vi "Marquee.vi"(8 "Indicator or ctrl to look up value change":refnum<vi>, 9 "Iteration":i8, 10 "error in (no error)":errorcluster, 11 "Text":string) -> (2 "error out":errorcluster, 3 "shutdown":bool=TRUE)   [LabVIEW 2021]
doc: "Showing marquee animation"
uses:
  System.Windows.Forms
panel:
  in  "Panel":refnum<k24>(container) caption="Closing WebSDR Cat-Control...."
  in  "stop":bool
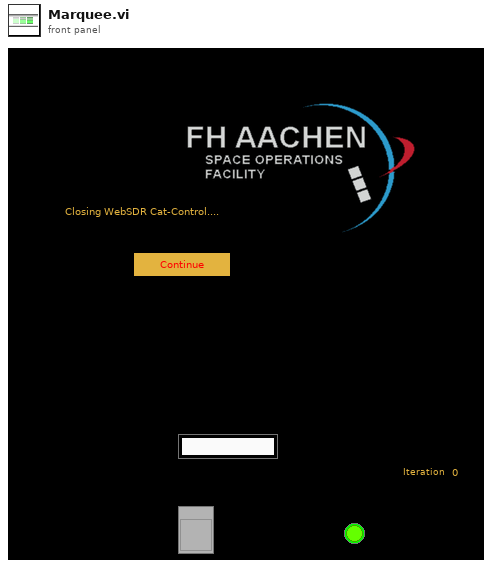
[diagram p1: front panel]
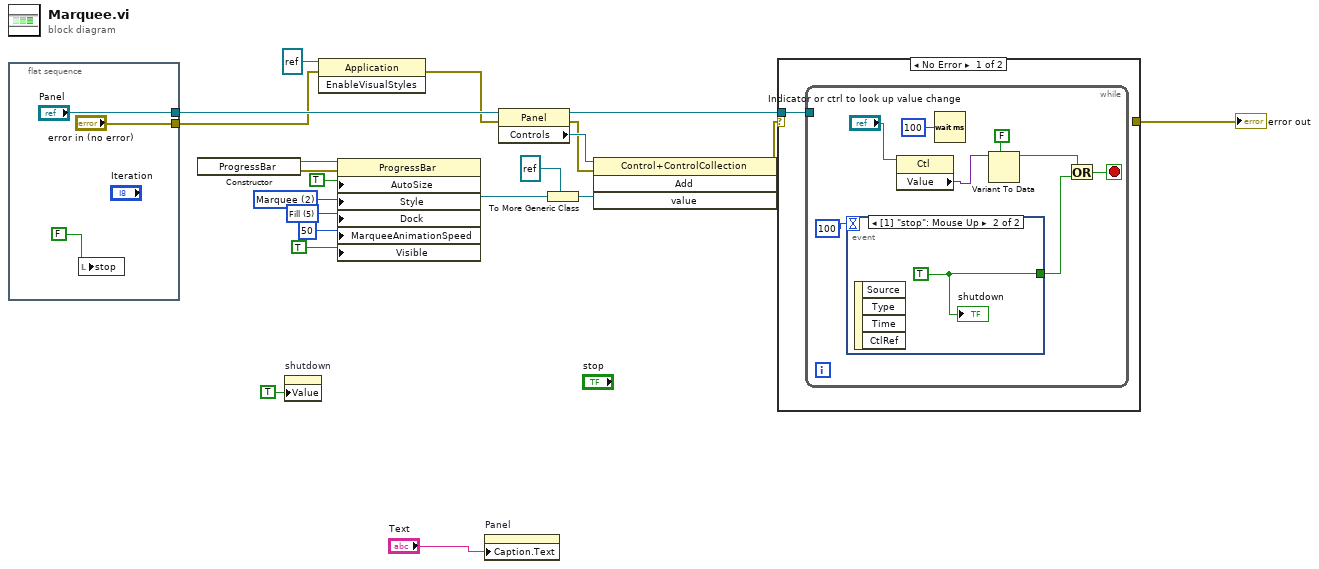
[diagram p0: block diagram]
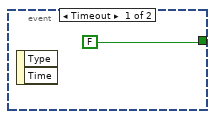
[diagram p2: hidden frame]
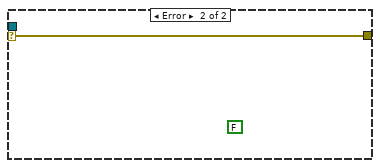
[diagram p3: hidden frame]
diagram:
  w16 = 5 items=["None", "Top", "Bottom", "Left", "Right", "Fill"] ("Dock")
  w15 = 2 items=["Blocks", "Continuous", "Marquee"] ("Style")
  n1 = flat-sequence {
    tunnel: ["Panel"] -> w21
    tunnel: ["error in (no error)"] -> w4
    frame #0 {
      n2 = local write "stop"(FALSE ("ABORT?")) -> ()
    }
  }
  n3 = constructor class="ProgressBar"() -> (reference out=w12:refnum<k24>, error out=w14:errorcluster)  [unwired: 3 in, 1 out]
  n4 = property on="shutdown" class="Bool (strict)"("Value"=TRUE ("shutdown")) -> ()  [unwired: 2 in, 2 out]
  n5 = invoke class="Application" method="EnableVisualStyles"(reference=refnum<k24> refnum ("new reference"), error in=w4) -> (error out=w3:errorcluster)  [unwired: 1 in, 2 out]
  n6 = property class="ProgressBar"(reference=w12, error in=w14, "AutoSize"=TRUE, "Style"=w15, "Dock"=w16, "MarqueeAnimationSpeed"=50, "Visible"=TRUE) -> (reference out=w8:refnum<k24>)  [unwired: 1 out]
  n7 = property on="Panel" class="AXCont"("Caption.Text"="Text") -> ()  [unwired: 2 in, 2 out]
  n8 = property class="Panel"(reference=w21, error in=w3) -> (reference out=w20:refnum<k24>, error out=w7:errorcluster, "Controls"=w11:refnum<k24>)
  n9 = To More Generic Class(target class=refnum<k24> refnum, reference=w8) -> (generic class reference=w9:refnum<k24>)
  n10 = invoke class="Control+ControlCollection" method="Add"(reference=w11, error in=w7, "value"=w9) -> (error out=w6:errorcluster)  [unwired: 1 in, 3 out]
  n11 = case shown="No Error" w6 {
    selector: w6 -> [_ w36]
    tunnel: w20 -> [w25 _]
    tunnel: [_ w36] -> w19
    frame No Error {
      n12 = while {
        tunnel: w25 -> [_]
        stop <- w31 stop-if-true
        n13 = event shown="[1] \"stop\": Mouse Up" {
          selector: _ -> [_ _]
          dyn-events: _ -> [_ _]
          timeout: 100 -> [_ _]
          tunnel: [FALSE w35] -> w30
          event Timeout {
            n14 = event-data() -> ()  [unwired: 3 out]
          }
          event "stop": Mouse Up {
            w35 = TRUE ("Boolean")
            n15 = event-data() -> ()  [unwired: 5 out]
            "shutdown" <- w35
          }
        }
        n16 = property on="Property Node" class="Ctl"(reference="Indicator or ctrl to look up value change") -> ("Value"=w27:variant)  [unwired: 1 in, 2 out]
        n17 = Wait (ms)(milliseconds to wait=u32 100) -> ()  [unwired: 1 out]
        n18 = Variant To Data(type=FALSE, Variant=w27) -> (data=w26:bool)  [unwired: 1 in, 1 out]
        n19 = Or(x=w26, y=w30) -> (x .or. y?=w31:bool)
      }
    }
    frame Error {
      (unwired) FALSE ("Boolean")
    }
  }
  "error out" <- w19
